vi "HT3_IntArrayToImgHeader.vi"(11 "Array":i32[](array[numeric])) -> (2 "PI Header":bool, 3 "Image Header":T1)   [LabVIEW 2013]
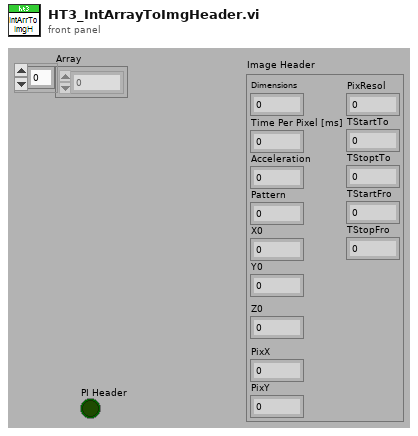
[diagram p1: front panel]
types:
  T1 = cluster{"Dimensions":i32, "Time Per Pixel [ms]":dbl, "Acceleration":i32, "Pattern":i32, "X0":sgl, "Y0":sgl, "Z0":dbl, "PixX":i32, "PixY":i32, "PixResol":sgl, "TStartTo":sgl, "TStoptTo":sgl, "TStartFro":sgl, "TStopFro":sgl}
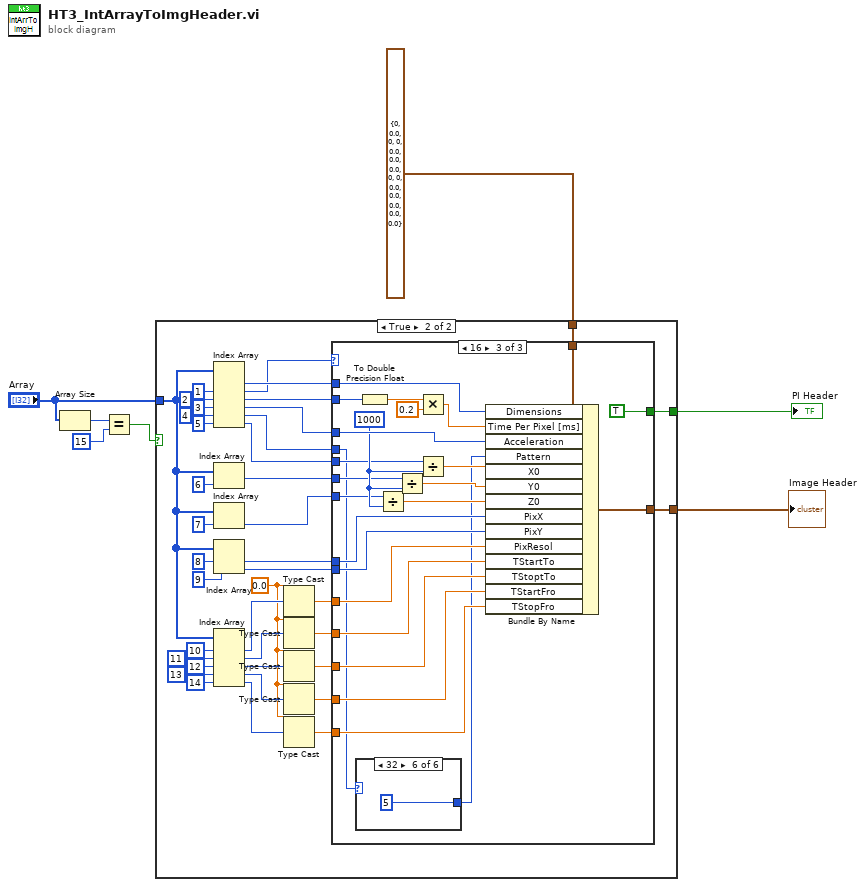
[diagram p0: block diagram]
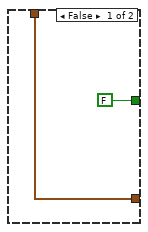
[diagram p2: hidden frame]
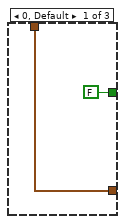
[diagram p3: hidden frame]
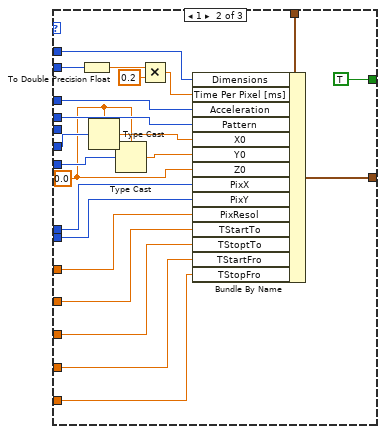
[diagram p4: hidden frame]
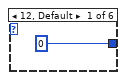
[diagram p5: hidden frame]
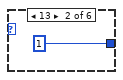
[diagram p6: hidden frame]
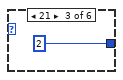
[diagram p7: hidden frame]
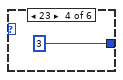
[diagram p8: hidden frame]
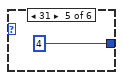
[diagram p9: hidden frame]
diagram:
  n1 = Array Size(array="Array") -> (size(s)=w6:i32)
  n2 = Equal?(x=w6, y=15) -> (x = y?=w4:bool)
  n3 = case shown="True" w4 {
    tunnel: "Array" -> [_ w39]
    tunnel: T1 {"Dimensions"=0, "Time Per Pixel [ms]"=0.0, "Acceleration"=0, "Pattern"=0, "X0"=0.0, "Y0"=0.0, "Z0"=0.0, "PixX"=0, "PixY"=0, "PixResol"=0.0, "TStartTo"=0.0, "TStoptTo"=0.0, "TStartFro"=0.0, "TStopFro"=0.0} ("Image Header") -> [w9 w33]
    tunnel: [w9 w32] -> w2
    tunnel: [FALSE w17] -> w1
    frame False {
    }
    frame True {
      w15 = sgl 0.0
      n4 = Index Array(array=w39, index #2=1 ("index"), index #3=2 ("index"), index #4=3 ("index"), index #5=4 ("index"), index #6=5 ("index")) -> (element #1=w31:i32, element #2=w16:i32, element #3=w30:i32, element #4=w10:i32, element #5=w11:i32, element #6=w12:i32)  [unwired: 1 in]
      n5 = Index Array(array=w39, index=6) -> (element=w13:i32)
      n6 = Index Array(array=w39, index=7) -> (element=w14:i32)
      n7 = Index Array(array=w39, index #1=8 ("index"), index #2=9 ("index")) -> (element #1=w29:i32, element #2=w28:i32)
      n8 = Index Array(array=w39, index #1=10 ("index"), index #2=11 ("index"), index #3=12 ("index"), index #4=13 ("index"), index #5=14 ("index")) -> (element #1=w27:i32, element #2=w26:i32, element #3=w25:i32, element #4=w23:i32, element #5=w24:i32)
      n9 = Type Cast(type=w15, x=w27) -> (*(type *) &x=w22:sgl)
      n10 = Type Cast(type=w15, x=w26) -> (*(type *) &x=w19:sgl)
      n11 = Type Cast(type=w15, x=w25) -> (*(type *) &x=w20:sgl)
      n12 = Type Cast(type=w15, x=w23) -> (*(type *) &x=w18:sgl)
      n13 = Type Cast(type=w15, x=w24) -> (*(type *) &x=w21:sgl)
      n14 = case shown="16" w16 {
        tunnel: w33 -> [w50 w72 w97]
        tunnel: [w50 w71 w96] -> w32
        tunnel: w31 -> [_ w70 w95]
        tunnel: w30 -> [_ w69 w94]
        tunnel: w10 -> [_ w65 w90]
        tunnel: w11 -> [_ w64 w74]
        tunnel: w13 -> [_ w54 w76]
        tunnel: w14 -> [_ w52 w77]
        tunnel: w29 -> [_ w63 w89]
        tunnel: w28 -> [_ w62 w88]
        tunnel: w22 -> [_ w61 w87]
        tunnel: w21 -> [_ w60 w86]
        tunnel: w20 -> [_ w59 w85]
        tunnel: w19 -> [_ w58 w84]
        tunnel: w18 -> [_ w57 w83]
        tunnel: [FALSE TRUE TRUE] -> w17
        tunnel: w12 -> [_ _ w75]
        frame 0, Default {
        }
        frame 1 {
          w51 = 0.0
          n15 = To Double Precision Float(number=w69) -> (double precision float=w68:dbl)
          n16 = Type Cast(type=w51, x=w54) -> (*(type *) &x=w55:dbl)
          n17 = Type Cast(type=w51, x=w52) -> (*(type *) &x=w53:dbl)
          n18 = Multiply(x=w68, y=0.2) -> (x*y=w66:dbl)
          n19 = Bundle By Name(cluster=w72, "Dimensions"=w70, "Time Per Pixel [ms]"=w66, "Acceleration"=w65, "Pattern"=w64, "X0"=w55, "Y0"=w53, "Z0"=w51, "PixX"=w63, "PixY"=w62, "PixResol"=w61, "TStartTo"=w58, "TStoptTo"=w59, "TStartFro"=w57, "TStopFro"=w60) -> (w71:T1)
        }
        frame 16 {
          w81 = 1000
          n20 = case shown="32" w74 {
            tunnel: [0 1 2 3 4 5] -> w73
            frame 12, Default {
            }
            frame 13 {
            }
            frame 21 {
            }
            frame 23 {
            }
            frame 31 {
            }
            frame 32 {
            }
          }
          n21 = To Double Precision Float(number=w94) -> (double precision float=w93:dbl)
          n22 = Divide(x=w77, y=w81) -> (x/y=w80:dbl)
          n23 = Divide(x=w76, y=w81) -> (x/y=w79:dbl)
          n24 = Multiply(x=w93, y=0.2) -> (x*y=w91:dbl)
          n25 = Divide(x=w75, y=w81) -> (x/y=w78:dbl)
          n26 = Bundle By Name(cluster=w97, "Dimensions"=w95, "Time Per Pixel [ms]"=w91, "Acceleration"=w90, "Pattern"=w73, "X0"=w78, "Y0"=w79, "Z0"=w80, "PixX"=w89, "PixY"=w88, "PixResol"=w87, "TStartTo"=w84, "TStoptTo"=w85, "TStartFro"=w83, "TStopFro"=w86) -> (w96:T1)
        }
      }
    }
  }
  "Image Header" <- w2
  "PI Header" <- w1
